vi "ClearDirectory.vi"(8 "error in (no error)":errorcluster, 11 "Directory in":path) -> (0 "error out":errorcluster, 3 "Directory out":path)   [LabVIEW 2017]
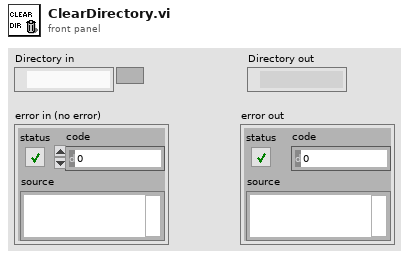
[diagram p1: front panel]
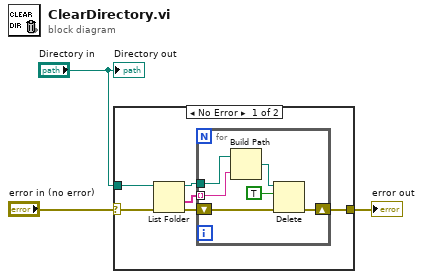
[diagram p0: block diagram]
diagram:
  n1 = case shown="No Error" "error in (no error)" {
    selector: "error in (no error)" -> [w9 w16]
    tunnel: "Directory in" -> [w8 _]
    tunnel: [w7 w16] -> w2
    frame No Error {
      n2 = List Folder(path=w8, error in=w9) -> (path out=w4:path, folder names=w5:string[], error out=w6:errorcluster)  [unwired: 2 in, 1 out]
      n3 = for {
        tunnel: w4 -> [w14]
        tunnel: w5 -> [w13] mode=indexing
        shift-right: [w10] -> w7
        shift-left: w6 -> [w11]
        n4 = Build Path(base path=w14, name or relative path=w13) -> (appended path=w12:path)
        n5 = Delete(path (use dialog)=w12, entire hierarchy (F)=TRUE, error in=w11) -> (error out=w10:errorcluster)  [unwired: 2 in, 2 out]
      }
    }
    frame Error {
    }
  }
  "error out" <- w2
  "Directory out" <- "Directory in"
